vi "HW_7p1_Task3_PRADHASK.vi"() -> ()   [LabVIEW 2016]
uses:
  <vilib>/express/express arith-compare/Formula/XNode/ExpressFormulaBlockNode.xnode
panel:
  out "Percentage bad":dbl
  in  "Num of trial expt to run":dbl
  in  "Current Tol (A)":dbl
  in  "Voltage (V)":dbl
  in  "Resistor tol":dbl
  in  "Resistor val (ohm)":dbl
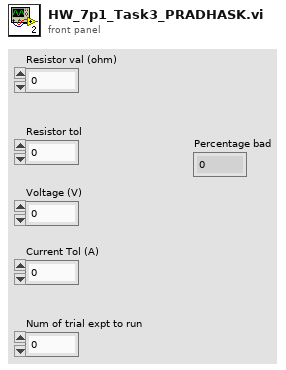
[diagram p1: front panel]
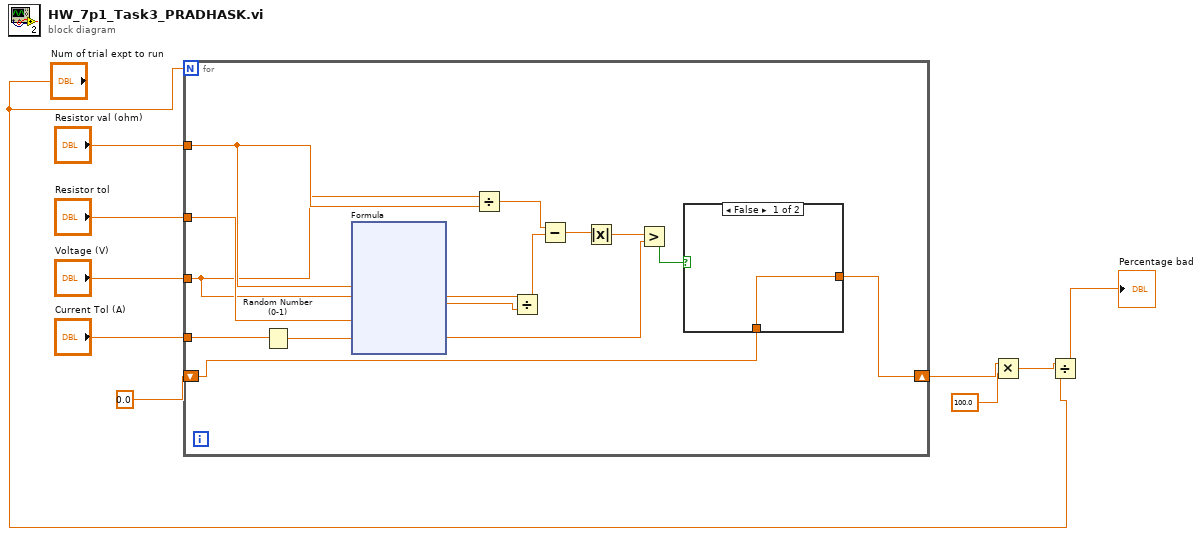
[diagram p0: block diagram]
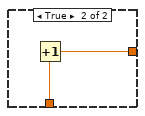
[diagram p2: hidden frame]
diagram:
  n1 = for {
    N: "Num of trial expt to run" -> [_]
    tunnel: "Resistor tol" -> [w23]
    tunnel: "Voltage (V)" -> [w19]
    tunnel: "Resistor val (ohm)" -> [w21]
    tunnel: "Current Tol (A)" -> [w15]
    shift-right: [w11] -> w4
    shift-left: 0.0 -> [w12]
    n2 = Random Number (0-1)() -> (number: 0 to 1=w22:dbl)
    n3 = xnode "Formula"("R"=w21, "Tol"=w23, "RND"=w22) -> ("Result"=w20:dbl)  [unwired: 1 in, 1 out]
    n4 = Divide(x=w19, y=w21) -> (x/y=w18:dbl)
    n5 = Divide(x=w19, y=w20) -> (x/y=w17:dbl)
    n6 = Subtract(x=w18, y=w17) -> (x-y=w16:dbl)
    n7 = Absolute Value(x=w16) -> (abs(x)=w14:dbl)
    n8 = Greater?(x=w14, y=w15) -> (0:w13:bool)
    n9 = case shown="False" w13 {
      tunnel: w12 -> [w24 w26]
      tunnel: [w24 w25] -> w11
      frame False {
      }
      frame True {
        n10 = Increment(x=w26) -> (x+1=w25:dbl)
      }
    }
  }
  n11 = Multiply(x=w4, y=100.0) -> (x*y=w6:dbl)
  n12 = Divide(x=w6, y="Num of trial expt to run") -> (x/y=→"Percentage bad":dbl)
